vi "Read 2ndStrikerPositioned.vi"(8 "error in (no error)":errorcluster, 11 "PreparePassPlay in":refnum<class "PreparePassPlay.lvclass">) -> (0 "error out":errorcluster, 2 "2ndStrikerPositioned":bool, 3 "PreparePassPlay out":refnum<class "PreparePassPlay.lvclass">)   [LabVIEW 2023, in "PreparePassPlay.lvclass"]
uses:
  PreparePassPlay.lvclass
  PreparePassPlay.lvclass/PreparePassPlay.ctl
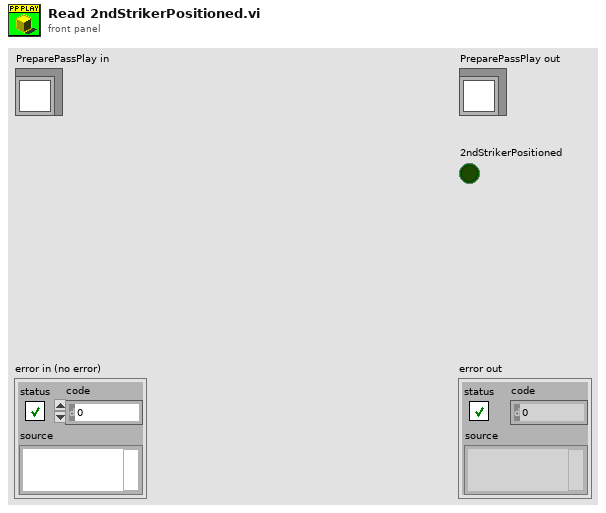
[diagram p1: front panel]
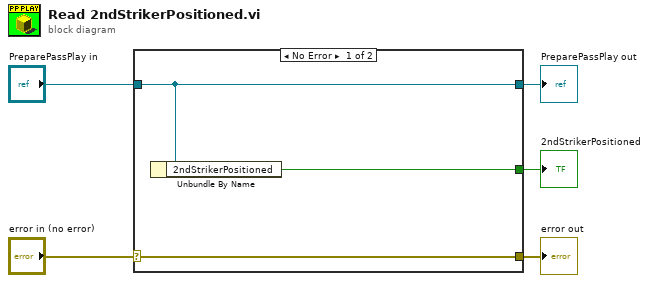
[diagram p0: block diagram]
diagram:
  n1 = case shown="No Error" "error in (no error)" {
    selector: "error in (no error)" -> [w8 w9]
    tunnel: [w8 w9] -> w4
    tunnel: [w7 w10] -> w2
    tunnel: "PreparePassPlay in" -> [w7 w10]
    tunnel: [w6 _] -> w1
    frame No Error {
      n2 = Unbundle By Name(w7) -> ("2ndStrikerPositioned"=w6:bool)
    }
    frame Error {
    }
  }
  "error out" <- w4
  "PreparePassPlay out" <- w2
  "2ndStrikerPositioned" <- w1
